vi "Stop Nodes.vi"(8 "error in (no error)":errorcluster, 11 "Server in":refnum<class "Server.lvclass">) -> (0 "error out":errorcluster, 3 "Server out":refnum<class "Server.lvclass">)   [LabVIEW 2013, in "JKI_Python_Bridge_for_LV.lvlib" / "Server.lvclass"]
uses:
  Server.lvclass
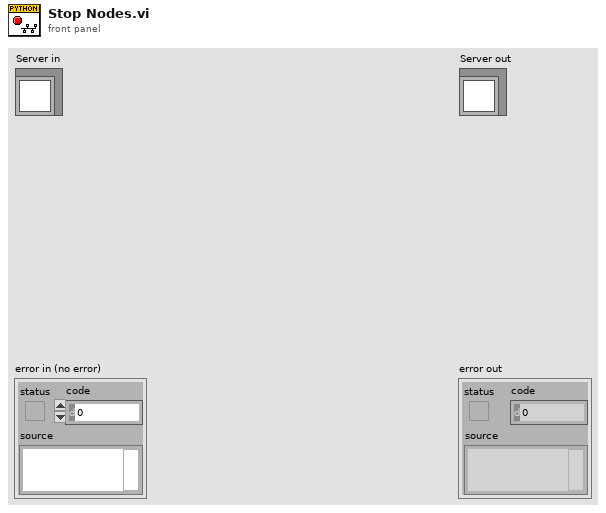
[diagram p1: front panel]
types:
  T1 = typedef "JKI_Python_Bridge_for_LV.lvlib/Server.lvclass/Public Events - Cluster.ctl" = cluster{"Stop Nodes":refnum<user-event>}
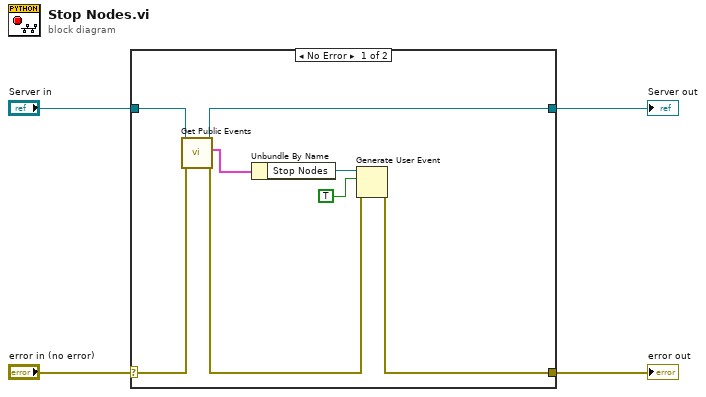
[diagram p0: block diagram]
diagram:
  n1 = case shown="No Error" "error in (no error)" {
    selector: "error in (no error)" -> [w10 w14]
    tunnel: [w6 w14] -> w3
    tunnel: [w11 w13] -> w1
    tunnel: "Server in" -> [w12 w13]
    frame No Error {
      n2 = call "Get Public Events.vi"("error in (no error)"=w10, "JKI_Python_Server in"=w12) -> ("error out"=w7:errorcluster, "Public Events"=w9:T1, "JKI_Python_Server out"=w11:refnum<class "Server.lvclass">)  [unwired: 7 in]
      n3 = Unbundle By Name(w9) -> ("Stop Nodes"=w8:refnum<user-event>)
      n4 = Generate User Event(user event=w8, event data cluster=TRUE ("event data"), error in=w7) -> (error out=w6:errorcluster)  [unwired: 1 in, 1 out]
    }
    frame Error {
    }
  }
  "error out" <- w3
  "Server out" <- w1
